vi "sCMOS_read_extract_images.vi"(4 "ROI":T2, 6 "error in":errorcluster, 7 "Image contrast":cluster{i32, i32}(slide) scale=0.0..16000.0, 8 "ROI IN":T1, 9 "Contrast IN":T1, 10 "Image":T1) -> (0 "error out":errorcluster, 1 "ROI OUT":T1, 2 "Contrast OUT":T1, 3 "Intensity range":T3)   [LabVIEW 2015]
uses:
  <vilib>/vision/Image Controls.llb/IMAQ Image.ctl
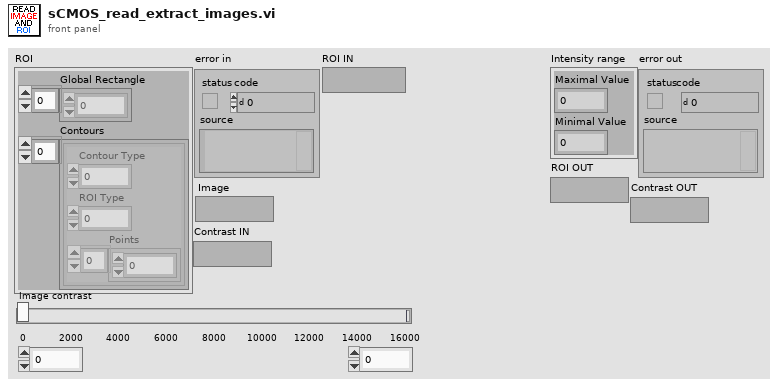
[diagram p1: front panel]
types:
  T1 = typedef "IMAQ Image.ctl" = refnum<image>
  T2 = cluster{"Global Rectangle":i32[], "Contours":cluster{"Contour Type":u32, "ROI Type":u32, "Points":i32[]}[]}
  T3 = cluster{"Maximal Value":sgl, "Minimal Value":sgl}
  T4 = cluster{"Mean Value":sgl, "Standard Variation":sgl, "Minimal Value":sgl, "Maximal Value":sgl, "Area (calibrated)":sgl, "Area (pixels)":u32, "%":sgl, "Calibration Valid":bool}
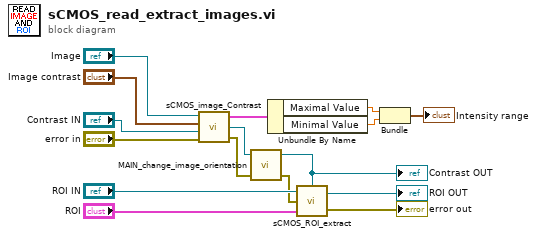
[diagram p0: block diagram]
diagram:
  n1 = call "sCMOS_image_Contrast.vi"("error in"="error in", "Image Dst"="Contrast IN", "Image contrast"="Image contrast", "New Image"="Image") -> ("error out"=w4:errorcluster, "Image Dst Out"=w3:T1, "Global Report"=w15:T4)
  n2 = call "MAIN_change_image_orientation.vi"("error in"=w4, "Image IN"=w3) -> ("error out"=w1:errorcluster, "Image Out"=w2:T1)  [unwired: 2 in]
  "Contrast OUT" <- w2
  n3 = Unbundle By Name(w15) -> ("Maximal Value"=w14:sgl, "Minimal Value"=w13:sgl)
  n4 = call "sCMOS_ROI_extract.vi"("Image IN"=w2, "ROI"="ROI", "error in"=w1, "Image ROI"="ROI IN") -> ("error out"=→"error out":errorcluster, "Image Out"=→"ROI OUT":T1)
  n5 = Bundle("Maximal Value"=w14, "Minimal Value"=w13) -> (→"Intensity range":T3)  [unwired: 1 in]
